vi "Autonomous Independent.vi"   [LabVIEW 2017]
doc: "This VI is called when autonomous begins, and will automatically be terminated when autonomous ends. You can carry out timed or sensor driven robot movement independently without needing to return to the caller."
uses:
  <vilib>/Rock Robotics/WPI/Solenoid/WPI_SolenoidValue.ctl
  <vilib>/Rock Robotics/Network Tables/NT Read String.vi
  <vilib>/Rock Robotics/WPI/Utilities/WPI_GetSetVariantRefNum.vi
  <vilib>/Rock Robotics/Network Tables/NT Write Numeric Array.vi
  <vilib>/Rock Robotics/WPI/Solenoid/WPI_SolenoidSetEnum.vi
panel:
  # "Be sure to right-click and choose Data Operations>>Make Current Value default if you want to save the array values with the VI"
types:
  T1 = typedef "WPI_JoystickDevRef.ctl" = cluster{"Device":T2}
  T2 = typedef "WPI_JoystickDeviceEnum.ctl" = enum16{"USB 0", "USB 1", "USB 2", "USB 3", "USB 4", "USB 5"}
  T3 = typedef "WPI_SolenoidDevRef.ctl" = cluster{"DevStatus":errorcluster, "Pneumatics Control Module":u8, "Forward Solenoid Channel":T4, "Reverse Solenoid Channel":T4}
  T4 = typedef "WPI_SolenoidChannel.ctl" = enum8{"Solenoid 0", "Solenoid 1", "Solenoid 2", "Solenoid 3", "Solenoid 4", "Solenoid 5", "Solenoid 6", "Solenoid 7", "Invalid"}
  T5 = typedef "WPI_MotorControlDeviceRef.ctl" = cluster{"DeviceStatus":errorcluster, "Type":T6, "PWM":cluster{"PWM Channel":T7, "DeadBand":T8}, "CAN":cluster{"Device Number":u8, "SetOutput VI Ref":variant, "GetOutput VI Ref":variant, "Enable VI Ref":variant, "Disable VI Ref":variant, "Data":variant}, "Invert":bool, "DIO PWM":cluster{"PWM \"Enable\" Channel":T7, "DIOChannel":T9, "PWM Rate":dbl}}
  T6 = typedef "WPI_MotorControlType.ctl" = enum16{"PWM", "CAN", "DIO PWM"}
  T7 = typedef "FPGA_DIOPWMChannel.ctl" = enum8{"PWM 0", "PWM 1", "PWM 2", "PWM 3", "PWM 4", "PWM 5", "PWM 6", "PWM 7", "PWM 8", "PWM 9", "PWM MXP 0", "PWM MXP 1", "PWM MXP 2", "PWM MXP 3", "PWM MXP 4", "PWM MXP 5", "PWM MXP 6", "PWM MXP 7", "PWM MXP 8", "PWM MXP 9", "Invalid"}
  T8 = typedef "WPI_PWMDeadband.ctl" = cluster{"Name":string, "maxPositivePwm":i32, "minPositivePwm":i32, "centerPwm":i32, "maxNegativePwm":i32, "minNegativePwm":i32, "angularRange":u16}
  T9 = typedef "FPGA_DIOChannel.ctl" = enum8{"DIO 0", "DIO 1", "DIO 2", "DIO 3", "DIO 4", "DIO 5", "DIO 6", "DIO 7", "DIO 8", "DIO 9", "DIO MXP 0", "DIO MXP 1", "DIO MXP 2", "DIO MXP 3", "DIO MXP 4", "DIO MXP 5", "DIO MXP 6", "DIO MXP 7", "DIO MXP 8", "DIO MXP 9", "DIO MXP 10", "DIO MXP 11", "DIO MXP 12", "DIO MXP 13", "DIO MXP 14", "DIO MXP 15", "SPI Port CS1", "SPI Port CS2", "SPI Port CS3", "SPI Port MISO", "SPI Port MOSI", "Invalid"}
  T10 = typedef "WPI_RobotDriveDevRef.ctl" = cluster{"DevStatus":errorcluster, "Motors[]":T5[], "Square Inputs":bool, "Max Output":dbl}
  T11 = typedef "WPI_SolenoidValue.ctl" = enum16{"Off", "On", "Forward", "Reverse"}
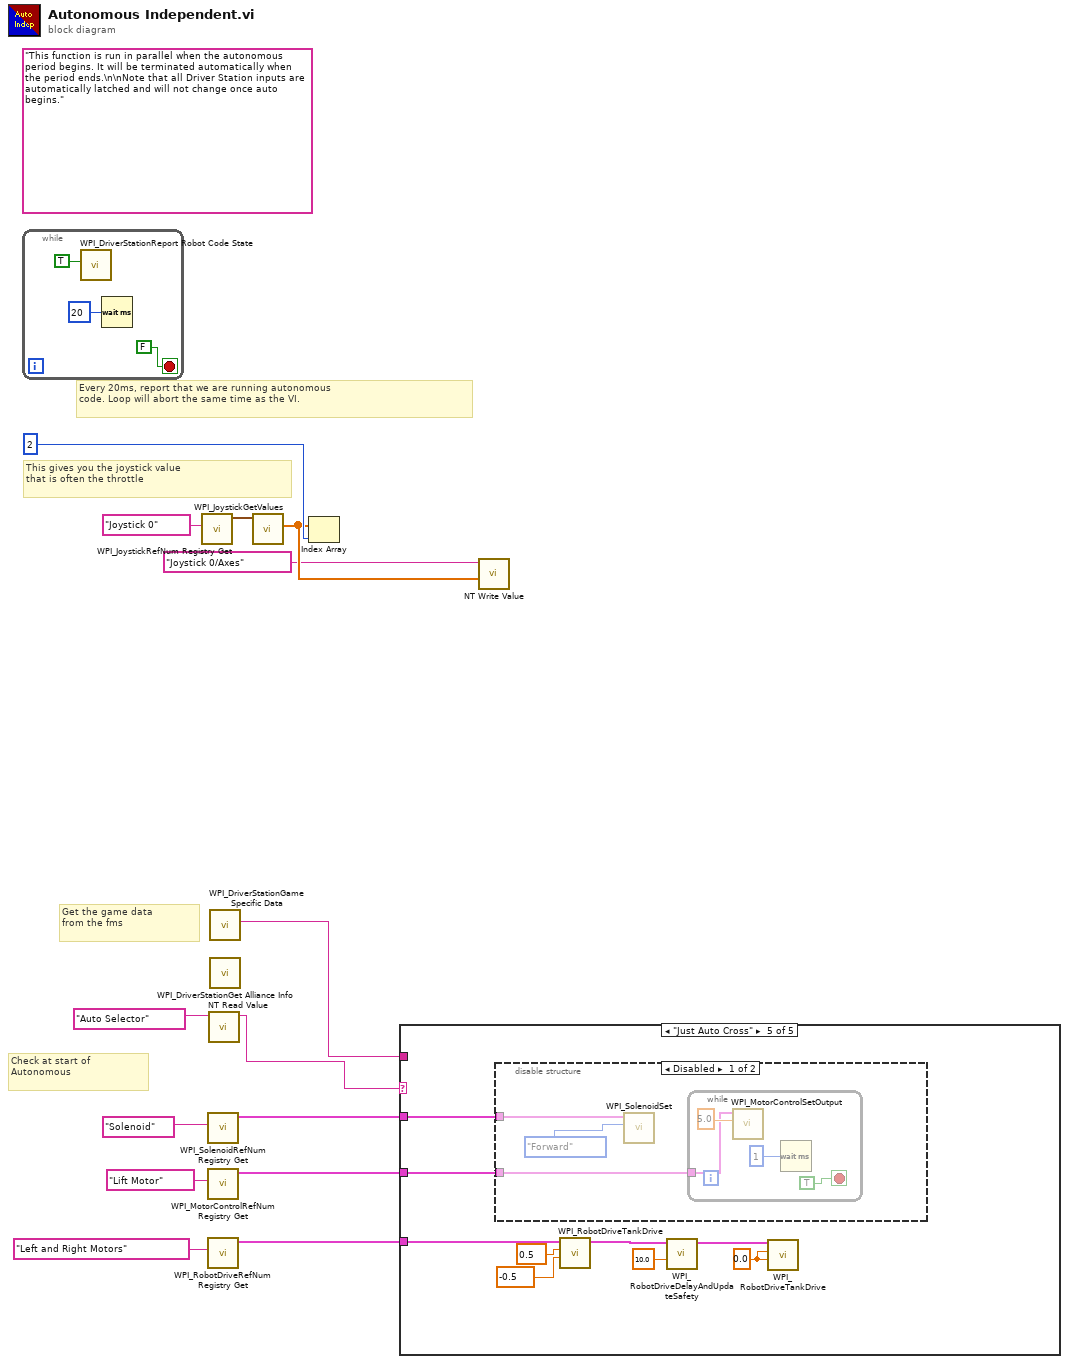
[diagram p0: block diagram]
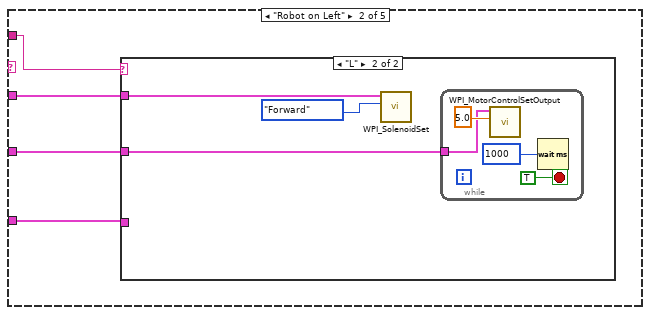
[diagram p3: hidden frame]
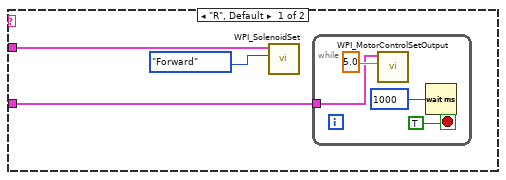
[diagram p4: hidden frame]
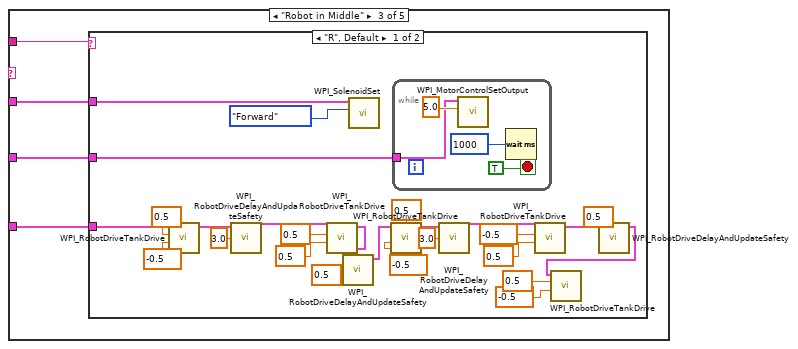
[diagram p5: hidden frame]
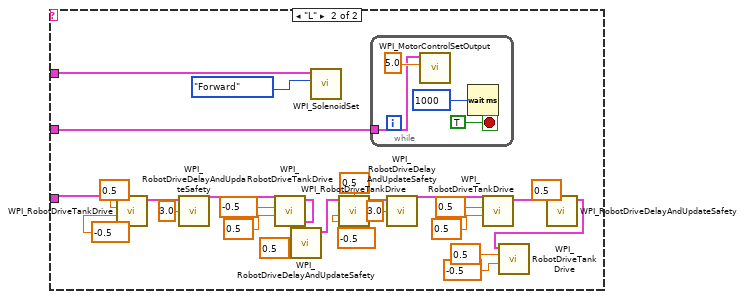
[diagram p6: hidden frame]
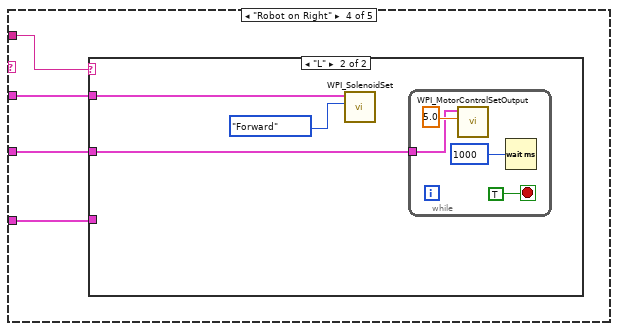
[diagram p7: hidden frame]
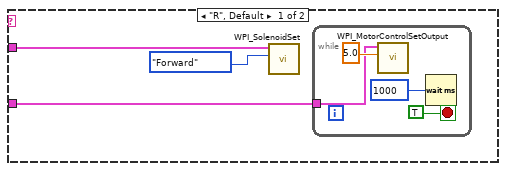
[diagram p8: hidden frame]
diagram:
  (unwired) "This function is run in parallel when the autonomous period begins. It will be terminated automatically when the period ends.\n\nNote that all Driver Station inputs are automatically latched and will not change once auto begins."
  # "Get the game data\nfrom the fms"
  # "This gives you the joystick value\nthat is often the throttle"
  # "Check at start of\nAutonomous"
  # "Every 20ms, report that we are running autonomous\ncode. Loop will abort the same time as the VI."
  n1 = while {
    stop <- FALSE stop-if-true
    n2 = call <vilib>:"WPI_DriverStationReport Robot Code State.vi"("Autonomous"=TRUE) -> ()  [unwired: 10 in, 1 out]
    n3 = Wait (ms)(milliseconds to wait=u32 20) -> ()  [unwired: 1 out]
  }
  n4 = call <vilib>:"WPI_JoystickRefNum Registry Get.vi"("refnum name"="Joystick 0") -> ("JoystickDevRef"=w8:T1)  [unwired: 1 in, 9 out]
  n5 = call <vilib>:"WPI_SolenoidRefNum Registry Get.vi"("refnum name"="Solenoid") -> ("SolenoidDevRef"=w3:T3)  [unwired: 9 in, 1 out]
  n6 = call <vilib>:"WPI_MotorControlRefNum Registry Get.vi"("refnum name"="Lift Motor") -> ("MotorControlDevRef"=w1:T5)  [unwired: 9 in, 1 out]
  n7 = call <vilib>:"WPI_RobotDriveRefNum Registry Get.vi"("refnum name"="Left and Right Motors") -> ("RobotDriveDevRef"=w11:T10)  [unwired: 1 in, 9 out]
  n8 = call-poly <vilib>:"NT Read Value.vi"("Name"="Auto Selector") -> ("String"=w13:string)  [unwired: 9 in, 1 out]
  n9 = call <vilib>:"WPI_DriverStationGame Specific Data.vi"() -> ("Game Specific Data"=w10:string)  [unwired: 11 in]
  n10 = call <vilib>:"WPI_DriverStationGet Alliance Info.vi"() -> ()  [unwired: 12 out]
  n11 = call <vilib>:"WPI_JoystickGetValues.vi"("JoystickDevRef"=w8) -> ("Axes"=w6:dbl[])  [unwired: 6 in, 4 out]
  n12 = Index Array(array=w6, index=2) -> ()  [unwired: 1 out]
  n13 = case shown="\"Just Auto Cross\"" w13 {
    tunnel: w11 -> [_ w18 w37 w101 w126]
    tunnel: w10 -> [_ w21 w36 w100 _]
    tunnel: w3 -> [_ w20 w39 w103 w125]
    tunnel: w1 -> [_ w19 w38 w102 w118]
    frame Default {
    }
    frame "Robot on Left" {
      n14 = case shown="\"L\"" w21 {
        tunnel: w20 -> [w23 w30]
        tunnel: w19 -> [w22 w29]
        tunnel: w18 -> [_ _]
        frame "R", Default {
          n15 = call-poly <vilib>:"WPI_SolenoidSet.vi"("Value"=WPI_SolenoidValue."Forward", "SolenoidDevRef"=w23) -> ()  [unwired: 8 in, 2 out]
          n16 = while {
            tunnel: w22 -> [w26]
            stop <- TRUE stop-if-true
            n17 = call <vilib>:"WPI_MotorControlSetOutput.vi"("Output"=5.0, "MotorControlDevRef"=w26) -> ()  [unwired: 7 in, 3 out]
            n18 = Wait (ms)(milliseconds to wait=u32 1000) -> ()  [unwired: 1 out]
          }
        }
        frame "L" {
          n19 = call-poly <vilib>:"WPI_SolenoidSet.vi"("Value"=WPI_SolenoidValue."Forward", "SolenoidDevRef"=w30) -> ()  [unwired: 8 in, 2 out]
          n20 = while {
            tunnel: w29 -> [w33]
            stop <- TRUE stop-if-true
            n21 = call <vilib>:"WPI_MotorControlSetOutput.vi"("Output"=5.0, "MotorControlDevRef"=w33) -> ()  [unwired: 7 in, 3 out]
            n22 = Wait (ms)(milliseconds to wait=u32 1000) -> ()  [unwired: 1 out]
          }
        }
      }
    }
    frame "Robot in Middle" {
      n23 = case shown="\"R\", Default" w36 {
        tunnel: w39 -> [w64 w89]
        tunnel: w38 -> [w63 w70]
        tunnel: w37 -> [w41 w88]
        frame "R", Default {
          n24 = call <vilib>:"WPI_RobotDriveTankDrive.vi"("Right axis value"=-0.5, "Left axis value"=0.5 ("X axis value"), "RobotDriveDevRef"=w41) -> ("RobotDriveDevRef"=w61:T10)  [unwired: 6 in, 2 out]
          n25 = call <vilib>:"WPI_RobotDriveDelayAndUpdateSafety.vi"("Delay (s)"=3.0, "RobotDriveDevRef"=w61) -> ("RobotDriveDevRef 2"=w62:T10)  [unwired: 8 in, 1 out]
          n26 = call <vilib>:"WPI_RobotDriveTankDrive.vi"("Right axis value"=0.5, "Left axis value"=0.5, "RobotDriveDevRef"=w62) -> ("RobotDriveDevRef"=w47:T10)  [unwired: 6 in, 2 out]
          n27 = call <vilib>:"WPI_RobotDriveDelayAndUpdateSafety.vi"("Delay (s)"=0.5, "RobotDriveDevRef"=w47) -> ("RobotDriveDevRef 2"=w46:T10)  [unwired: 8 in, 1 out]
          n28 = call-poly <vilib>:"WPI_SolenoidSet.vi"("Value"=WPI_SolenoidValue."Forward", "SolenoidDevRef"=w64) -> ()  [unwired: 8 in, 2 out]
          n29 = call <vilib>:"WPI_RobotDriveTankDrive.vi"("Right axis value"=-0.5, "Left axis value"=0.5 ("X axis value"), "RobotDriveDevRef"=w46) -> ("RobotDriveDevRef"=w55:T10)  [unwired: 6 in, 2 out]
          n30 = while {
            tunnel: w63 -> [w67]
            stop <- TRUE stop-if-true
            n31 = call <vilib>:"WPI_MotorControlSetOutput.vi"("Output"=5.0, "MotorControlDevRef"=w67) -> ()  [unwired: 7 in, 3 out]
            n32 = Wait (ms)(milliseconds to wait=u32 1000) -> ()  [unwired: 1 out]
          }
          n33 = call <vilib>:"WPI_RobotDriveDelayAndUpdateSafety.vi"("Delay (s)"=3.0, "RobotDriveDevRef"=w55) -> ("RobotDriveDevRef 2"=w56:T10)  [unwired: 8 in, 1 out]
          n34 = call <vilib>:"WPI_RobotDriveTankDrive.vi"("Right axis value"=0.5, "Left axis value"=-0.5, "RobotDriveDevRef"=w56) -> ("RobotDriveDevRef"=w50:T10)  [unwired: 6 in, 2 out]
          n35 = call <vilib>:"WPI_RobotDriveDelayAndUpdateSafety.vi"("Delay (s)"=0.5, "RobotDriveDevRef"=w50) -> ("RobotDriveDevRef 2"=w44:T10)  [unwired: 8 in, 1 out]
          n36 = call <vilib>:"WPI_RobotDriveTankDrive.vi"("Right axis value"=-0.5, "Left axis value"=0.5, "RobotDriveDevRef"=w44) -> ()  [unwired: 6 in, 3 out]
        }
        frame "L" {
          n37 = call <vilib>:"WPI_RobotDriveTankDrive.vi"("Right axis value"=-0.5, "Left axis value"=0.5 ("X axis value"), "RobotDriveDevRef"=w88) -> ("RobotDriveDevRef"=w94:T10)  [unwired: 6 in, 2 out]
          n38 = call <vilib>:"WPI_RobotDriveDelayAndUpdateSafety.vi"("Delay (s)"=3.0, "RobotDriveDevRef"=w94) -> ("RobotDriveDevRef 2"=w95:T10)  [unwired: 8 in, 1 out]
          n39 = call <vilib>:"WPI_RobotDriveTankDrive.vi"("Right axis value"=0.5, "Left axis value"=-0.5, "RobotDriveDevRef"=w95) -> ("RobotDriveDevRef"=w76:T10)  [unwired: 6 in, 2 out]
          n40 = call <vilib>:"WPI_RobotDriveDelayAndUpdateSafety.vi"("Delay (s)"=0.5, "RobotDriveDevRef"=w76) -> ("RobotDriveDevRef 2"=w75:T10)  [unwired: 8 in, 1 out]
          n41 = call-poly <vilib>:"WPI_SolenoidSet.vi"("Value"=WPI_SolenoidValue."Forward", "SolenoidDevRef"=w89) -> ()  [unwired: 8 in, 2 out]
          n42 = call <vilib>:"WPI_RobotDriveTankDrive.vi"("Right axis value"=-0.5, "Left axis value"=0.5 ("X axis value"), "RobotDriveDevRef"=w75) -> ("RobotDriveDevRef"=w84:T10)  [unwired: 6 in, 2 out]
          n43 = while {
            tunnel: w70 -> [w97]
            stop <- TRUE stop-if-true
            n44 = call <vilib>:"WPI_MotorControlSetOutput.vi"("Output"=5.0, "MotorControlDevRef"=w97) -> ()  [unwired: 7 in, 3 out]
            n45 = Wait (ms)(milliseconds to wait=u32 1000) -> ()  [unwired: 1 out]
          }
          n46 = call <vilib>:"WPI_RobotDriveDelayAndUpdateSafety.vi"("Delay (s)"=3.0, "RobotDriveDevRef"=w84) -> ("RobotDriveDevRef 2"=w85:T10)  [unwired: 8 in, 1 out]
          n47 = call <vilib>:"WPI_RobotDriveTankDrive.vi"("Right axis value"=0.5, "Left axis value"=0.5, "RobotDriveDevRef"=w85) -> ("RobotDriveDevRef"=w79:T10)  [unwired: 6 in, 2 out]
          n48 = call <vilib>:"WPI_RobotDriveDelayAndUpdateSafety.vi"("Delay (s)"=0.5, "RobotDriveDevRef"=w79) -> ("RobotDriveDevRef 2"=w73:T10)  [unwired: 8 in, 1 out]
          n49 = call <vilib>:"WPI_RobotDriveTankDrive.vi"("Right axis value"=-0.5, "Left axis value"=0.5, "RobotDriveDevRef"=w73) -> ()  [unwired: 6 in, 3 out]
        }
      }
    }
    frame "Robot on Right" {
      n50 = case shown="\"L\"" w100 {
        tunnel: w103 -> [w105 w112]
        tunnel: w102 -> [w104 w111]
        tunnel: w101 -> [_ _]
        frame "R", Default {
          n51 = call-poly <vilib>:"WPI_SolenoidSet.vi"("Value"=WPI_SolenoidValue."Forward", "SolenoidDevRef"=w105) -> ()  [unwired: 8 in, 2 out]
          n52 = while {
            tunnel: w104 -> [w108]
            stop <- TRUE stop-if-true
            n53 = call <vilib>:"WPI_MotorControlSetOutput.vi"("Output"=5.0, "MotorControlDevRef"=w108) -> ()  [unwired: 7 in, 3 out]
            n54 = Wait (ms)(milliseconds to wait=u32 1000) -> ()  [unwired: 1 out]
          }
        }
        frame "L" {
          n55 = call-poly <vilib>:"WPI_SolenoidSet.vi"("Value"=WPI_SolenoidValue."Forward", "SolenoidDevRef"=w112) -> ()  [unwired: 8 in, 2 out]
          n56 = while {
            tunnel: w111 -> [w115]
            stop <- TRUE stop-if-true
            n57 = call <vilib>:"WPI_MotorControlSetOutput.vi"("Output"=5.0, "MotorControlDevRef"=w115) -> ()  [unwired: 7 in, 3 out]
            n58 = Wait (ms)(milliseconds to wait=u32 1000) -> ()  [unwired: 1 out]
          }
        }
      }
    }
    frame "Just Auto Cross" {
      w119 = 0.0 ("X axis value")
      n59 = disable-structure shown="Disabled" {
        disable-tunnel: w125 -> [w129 _]
        disable-tunnel: w118 -> [w127 _]
        frame Disabled {
          n60 = call-poly <vilib>:"WPI_SolenoidSet.vi"("Value"=WPI_SolenoidValue."Forward", "SolenoidDevRef"=w129) -> ()  [unwired: 8 in, 2 out]
          n61 = while {
            tunnel: w127 -> [w131]
            stop <- TRUE stop-if-true
            n62 = call <vilib>:"WPI_MotorControlSetOutput.vi"("Output"=5.0, "MotorControlDevRef"=w131) -> ()  [unwired: 7 in, 3 out]
            n63 = Wait (ms)(milliseconds to wait=u32 1) -> ()  [unwired: 1 out]
          }
        }
        frame Enabled {
        }
      }
      n64 = call <vilib>:"WPI_RobotDriveTankDrive.vi"("Right axis value"=-0.5, "Left axis value"=0.5 ("X axis value"), "RobotDriveDevRef"=w126) -> ("RobotDriveDevRef"=w123:T10)  [unwired: 6 in, 2 out]
      n65 = call <vilib>:"WPI_RobotDriveDelayAndUpdateSafety.vi"("Delay (s)"=10.0, "RobotDriveDevRef"=w123) -> ("RobotDriveDevRef 2"=w124:T10)  [unwired: 8 in, 1 out]
      n66 = call <vilib>:"WPI_RobotDriveTankDrive.vi"("Right axis value"=w119, "Left axis value"=w119, "RobotDriveDevRef"=w124) -> ()  [unwired: 6 in, 3 out]
    }
  }
  n67 = call-poly <vilib>:"NT Write Value.vi"("Numeric Array"=w6, "Name"="Joystick 0/Axes") -> ()  [unwired: 9 in, 1 out]
